vi "Draw Text in Rect with Pixel Font.vi"(8 "string":string="Hello", 9 "Rectangle":T1, 11 "picture":picture) -> (3 "new picture":picture)   [LabVIEW 2021, in "Picture Pixel Fonts.lvlib"]
uses:
  <vilib>/LabVIEW Icon API/Pixel Fonts/Picture Pixel Fonts.lvlib
  <vilib>/LabVIEW Icon API/Pixel Fonts/Pixel Font/Pixel Font.lvlib
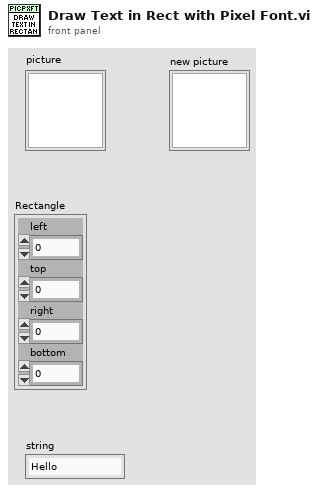
[diagram p1: front panel]
types:
  T1 = cluster{"left":i16, "top":i16, "right":i16, "bottom":i16}
  T2 = typedef "imagedata.ctl" = cluster{"image type":i32, "image depth":i32, "image":u8[], "mask":u8[], "colors":u32[], "Rectangle":cluster{"left":i16, "top":i16, "right":i16, "bottom":i16}}
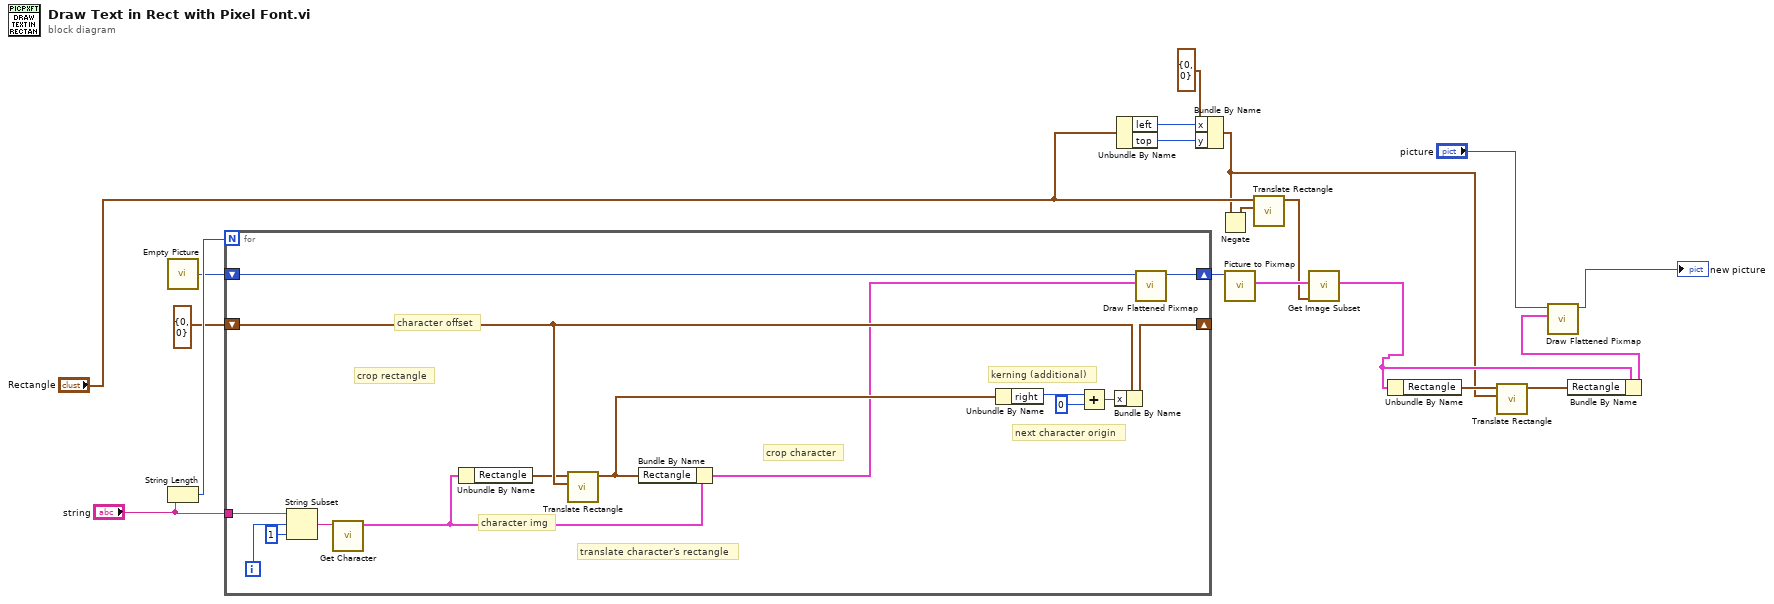
[diagram p0: block diagram]
diagram:
  n1 = call "Empty Picture"() -> ("empty picture"=w16:picture)
  n2 = String Length(string="string") -> (length=w18:i32)
  n3 = for {
    N: w18 -> [_]
    tunnel: "string" -> [w33]
    shift-right: [w23] -> _
    shift-left: cluster{"x":i16, "y":i16} {"x"=0, "y"=0} ("origin") -> [w25]
    shift-right: [w29] -> w14
    shift-left: w16 -> [w30]
    i -> [w31]
    # "crop rectangle"
    # "next character origin"
    # "translate character's rectangle"
    # "crop character"
    # "character img"
    # "character offset"
    # "kerning (additional)"
    n4 = String Subset(string=w33, offset (0)=w31, length (rest)=1 ("length (rest)")) -> (substring=w32:string)
    n5 = call <vilib>:"Get Character.vi"("string"=w32) -> ("image data"=w21:T2)  [unwired: 10 in]
    n6 = Unbundle By Name(w21) -> ("Rectangle"=w22:T1)
    n7 = call <vilib>:"Translate Rectangle.vi"("offset"=w25, "Rectangle in"=w22) -> ("Rectangle out"=w27:T1)  [unwired: 9 in]
    n8 = Bundle By Name(cluster=w21, "Rectangle"=w27) -> (w20:T2)
    n9 = Unbundle By Name(w27) -> ("right"=w26:i16)
    n10 = Add(x=w26, y=i16 0) -> (x+y=w24:i16)
    n11 = Bundle By Name(cluster=w25, "x"=w24) -> (w23:cluster{"x":i16, "y":i16})
    n12 = call <vilib>:"Draw Flattened Pixmap.vi"("image data"=w20, "picture"=w30) -> ("new picture"=w29:picture)  [unwired: 7 in]
  }
  n13 = Unbundle By Name("Rectangle") -> ("left"=w4:i16, "top"=w5:i16)
  n14 = Bundle By Name(cluster=cluster{"x":i16, "y":i16} {"x"=0, "y"=0} ("origin"), "x"=w4, "y"=w5) -> (w2:cluster{"x":i16, "y":i16})
  n15 = Negate(x=w2) -> (-x=w17:cluster{"x":i16, "y":i16})
  n16 = call <vilib>:"Picture to Pixmap.vi"("picture"=w14) -> ("image data"=w15:T2)  [unwired: 9 in, 1 out]
  n17 = call <vilib>:"Translate Rectangle.vi"("offset"=w17, "Rectangle in"="Rectangle") -> ("Rectangle out"=w11:T1)  [unwired: 9 in]
  n18 = call <vilib>:"Get Image Subset.vi"("subset rect"=w11, "image data"=w15) -> ("image subset"=w8:T2)  [unwired: 4 in, 1 out]
  n19 = Unbundle By Name(w8) -> ("Rectangle"=w10:T1)
  n20 = call <vilib>:"Translate Rectangle.vi"("offset"=w2, "Rectangle in"=w10) -> ("Rectangle out"=w9:T1)  [unwired: 9 in]
  n21 = Bundle By Name(cluster=w8, "Rectangle"=w9) -> (w7:T2)
  n22 = call <vilib>:"Draw Flattened Pixmap.vi"("image data"=w7, "picture"="picture") -> ("new picture"=→"new picture":picture)  [unwired: 7 in]
